vi "dfd_Validate Gain Settings.vi"(8 "error in (no error)":errorcluster, 10 "gain setting":T1={"gain processing target"=0, "gain wl"=16} {"gain processing target" items=["FXP Target", "Host"]}) -> (0 "error out":errorcluster, 2 "gain wl":i16)   [LabVIEW 2017, in "NI_DigFilter_FXP.lvlib"]
uses:
  <vilib>/addons/Digital Filter Design/NI_DigFilter_FXP.lvlib
  <vilib>/addons/Digital Filter Design/_Misc.llb/dfd_Error Handlers (Single).vi
  <vilib>/addons/Digital Filter Design/NI_DigFilterLicensed.lvlib
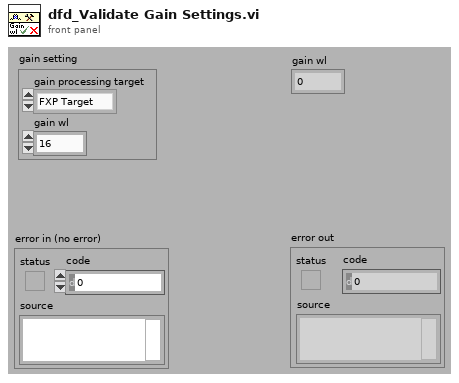
[diagram p1: front panel]
types:
  T1 = cluster{"gain processing target":u16, "gain wl":i16}
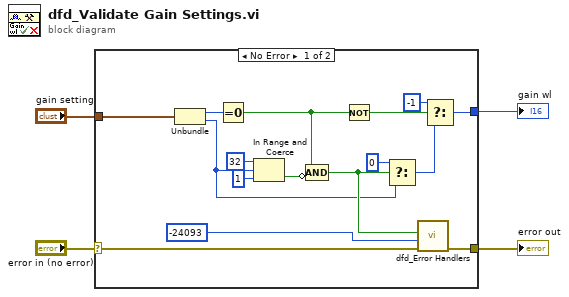
[diagram p0: block diagram]
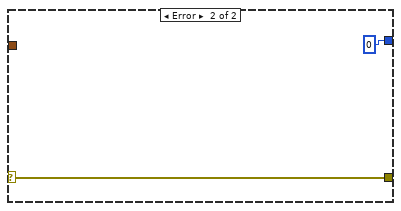
[diagram p2: hidden frame]
diagram:
  n1 = case shown="No Error" "error in (no error)" {
    selector: "error in (no error)" -> [w15 w21]
    tunnel: "gain setting" -> [w19 _]
    tunnel: [w13 w21] -> w2
    tunnel: [w11 i16 0 ("gain wl")] -> w1
    frame No Error {
      n2 = Unbundle(w19) -> ("gain processing target"=w20:u16, "gain wl"=w9:i16)
      n3 = Equal To 0?(x=w20) -> (x = 0?=w7:bool)
      n4 = In Range and Coerce(upper limit=i16 32, x=w9, lower limit=i16 1) -> (In Range?=w16:bool)  [unwired: 1 out]
      n5 = Compound Arithmetic op=AND(w7, invert w16) -> (w10:bool)
      n6 = Not(x=w7) -> (.not. x?=w6:bool)
      n7 = Select(t=i16 0, s=w10, f=w9) -> (s? t:f=w5:i16)
      n8 = call-poly <vilib>:"dfd_Error Handlers.vi"("error in (no error)"=w15, "error code"=-24093 ("ERR_INVALID_GAIN_SETTING"), "condition failed?"=w10) -> ("error out"=w13:errorcluster)  [unwired: 8 out]
      n9 = Select(t=i16 -1 ("f"), s=w6, f=w5) -> (s? t:f=w11:i16)
    }
    frame Error {
    }
  }
  "error out" <- w2
  "gain wl" <- w1
